vi "Exploracion.vi"() -> ()   [LabVIEW 2020]
uses:
  <vilib>/measure/NI_MABase.lvlib
panel:
  in  "Tab Control":enum32{"Temperatura", "Osciloscopio"}(tab)
  in  "Grabar Datos":bool
  in  "Temperatura gC":dbl(slide) scale=0.0..100.0
  out "Termometro gF":dbl(slide) scale=0.0..100.0
  in  "Limite":dbl
  out "Alarma":bool
  out "Supervisor":dynamicdata(graph)
  in  "Frecuencia":dbl(knob) scale=0.0..100.0
  in  "Amplitud":dbl(knob) scale=0.0..10.0
  out "Osciloscopio":waveform(dbl)(graph)
  in  "stop":bool
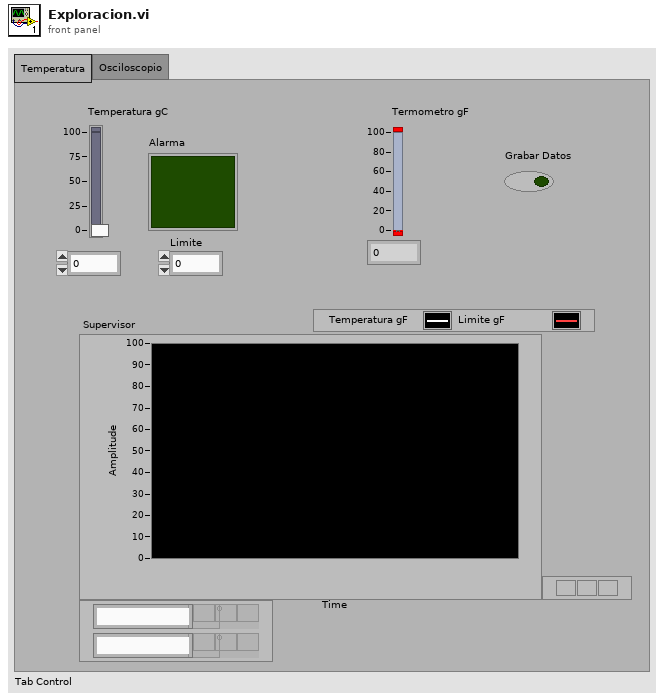
[diagram p1: front panel]
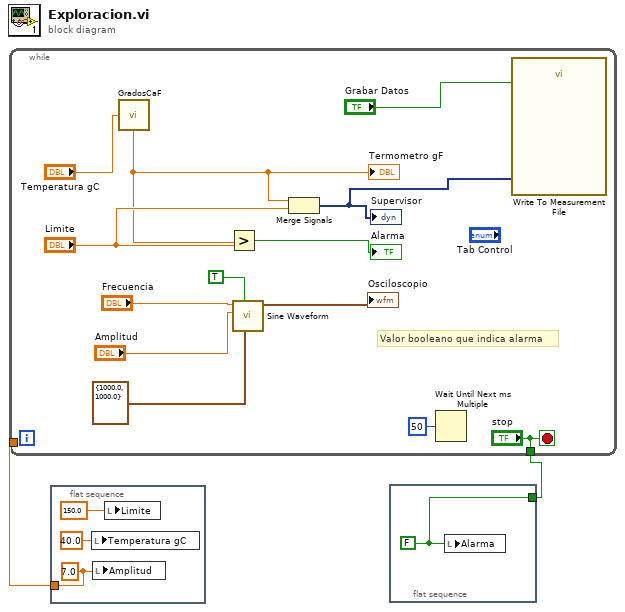
[diagram p0: block diagram]
diagram:
  n1 = while {
    tunnel: w2 -> [_]
    tunnel: ["stop"] -> w1
    stop <- "stop" stop-if-true
    # "Valor booleano que indica alarma"
    n2 = call "GradosCaF.vi"("Temperatura gC"="Temperatura gC") -> ("Temperatura gF"=w8:dbl)
    "Termometro gF" <- w8
    n3 = Greater?(x=w8, y="Limite") -> (0:→"Alarma":bool)
    n4 = call <vilib>:"Sine Waveform.vi"("sampling info"=cluster{"Fs":dbl, "#s":dbl} {"Fs"=1000.0, "#s"=1000.0}, "reset signal"=TRUE, "amplitude"="Amplitud", "frequency"="Frecuencia") -> ("signal out"=→"Osciloscopio":waveform(dbl))  [unwired: 6 in, 1 out]
    n5 = Merge Signals(w8, "Limite") -> (w3:dynamicdata)
    "Supervisor" <- w3
    n6 = Wait Until Next ms Multiple(millisecond multiple=u32 50) -> ()  [unwired: 1 out]
    n7 = call "Write To Measurement File"("Signals"=w3, "Enable"="Grabar Datos") -> ()  [unwired: 15 in, 3 out]
  }
  n8 = flat-sequence {
    tunnel: [w16] -> w2
    frame #0 {
      w16 = 7.0 ("Amplitud")
      n9 = local write "Temperatura gC"(40.0 ("Temperatura gC")) -> ()
      n10 = local write "Amplitud"(w16) -> ()
      n11 = local write "Limite"(150.0 ("Limite")) -> ()
    }
  }
  n12 = flat-sequence {
    tunnel: [w19] -> _
    tunnel: w1 -> [_]
    frame #0 {
      w19 = FALSE ("Alarma")
      n13 = local write "Alarma"(w19) -> ()
    }
  }
